vi "Configure Scripting Plugins.vi"() -> ()   [LabVIEW 2016]
uses:
  DQMH Scripting Plugins/PantherLAB Scripting Hooks/Controls or Constants--enum.ctl
  <resource>/dialog/lvconfig.llb/LV Config Read Boolean.vi
  <resource>/dialog/lvconfig.llb/LV Config Read Numeric (I32).vi
  <resource>/dialog/lvconfig.llb/LV Config Write Boolean.vi
  <resource>/dialog/lvconfig.llb/LV Config Write Numeric (I32).vi
  DQMH Scripting Plugins/PantherLAB Scripting Hooks/PantherLAB_Scripting.lvlib
panel:
  in  "wait for reply and timed out? terminals":bool
  in  "Create":T1
  in  "Create Controls/Indicators or Constants":bool
  in  "Panther Logs":bool
  # "If Enabled a fille called <PantherLAB_Log.csv> will be created next to the Active Project and a new row will be logged for all of these DQMH Actions:\n* Add New DQMH Module\n* Rename DQMH Module\n* Duplicate DQMH Module\n* Create New DQMH Event\n* Convert DQMH Event\n* Remove DQMH Event\n* Rename DQMH Event\n* Duplicate DQMH Event\n* Add Helper Looop to DQMH Module\n* Create RT Tester\n* New DQMH Unit Test"
  # "When the DQMH Framework creates a new DQMH Event, it automatically opens the Module's API Tester Block Diagram and it will add the 'Fire Event.vi'  for the new Event Created\n\nTo improve  the process of testing public events, this plugin will create controls and indicators or constants for every public request. You can also choose to include/Exclude the 'wait for reply (T)' and 'timed out?'"
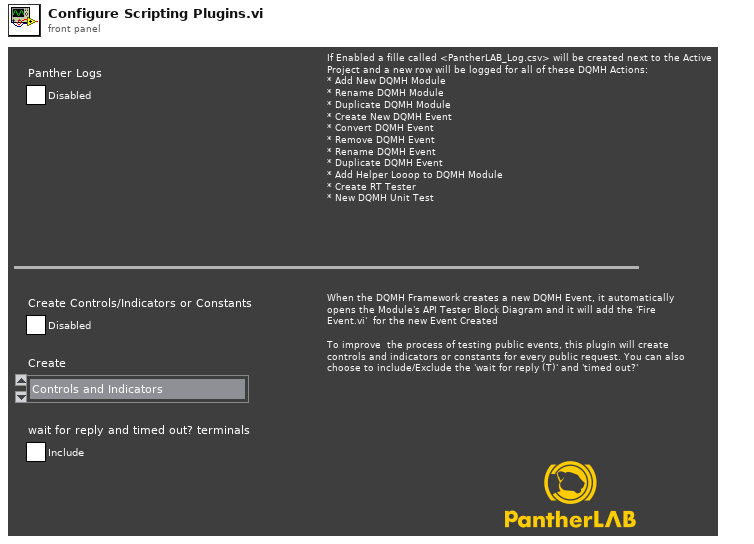
[diagram p1: front panel]
types:
  T1 = typedef "PantherLAB_Scripting.lvlib/Controls or Constants--enum.ctl" = enum16{"Controls and Indicators", "Constants and Indicators"}
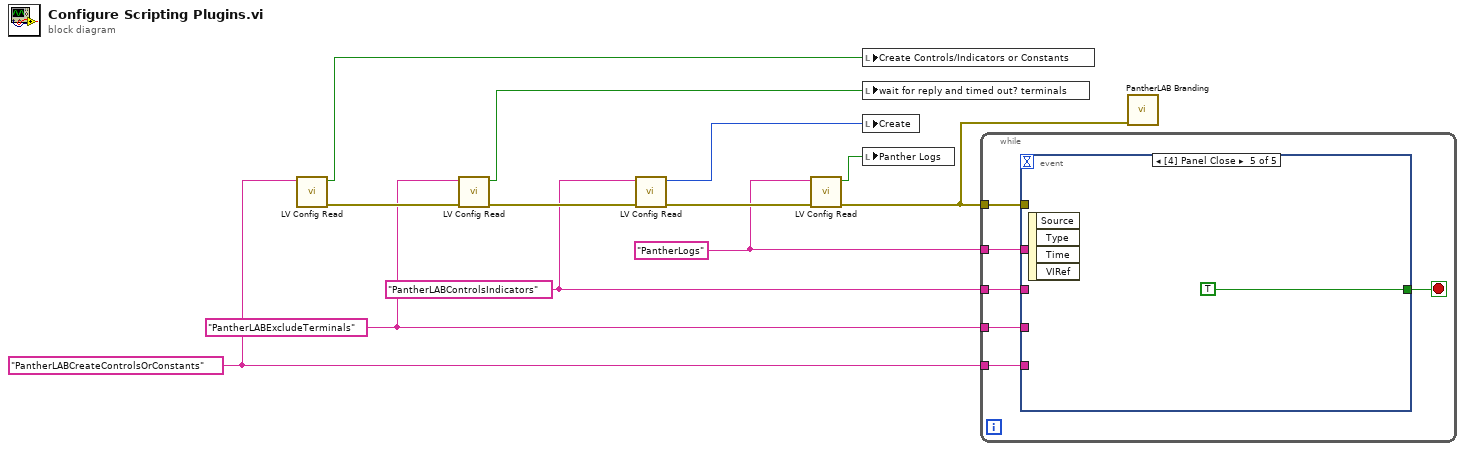
[diagram p0: block diagram]
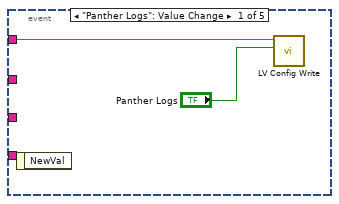
[diagram p2: hidden frame]
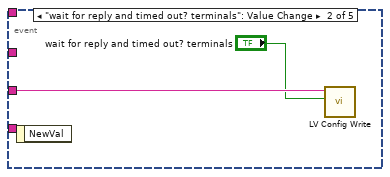
[diagram p3: hidden frame]
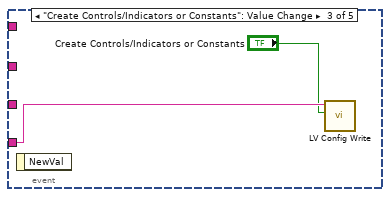
[diagram p4: hidden frame]
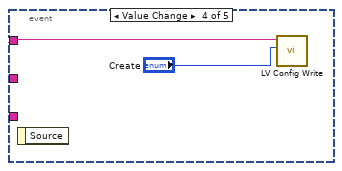
[diagram p5: hidden frame]
diagram:
  w2 = "PantherLABCreateControlsOrConstants" ("key")
  w3 = "PantherLABExcludeTerminals" ("key")
  w1 = "PantherLABControlsIndicators" ("key")
  w4 = "PantherLogs" ("key")
  n1 = call-poly <resource>:"LV Config Read.vi"("key"=w2) -> ("error out"=w10:errorcluster, "value"=w5:bool)  [unwired: 4 in, 1 out]
  n2 = call-poly <resource>:"LV Config Read.vi"("error in"=w10, "key"=w3) -> ("error out"=w11:errorcluster, "value"=w6:bool)  [unwired: 3 in, 1 out]
  n3 = call-poly <resource>:"LV Config Read.vi"("error in"=w11, "key"=w1) -> ("error out"=w12:errorcluster, "value"=w7:i32)  [unwired: 3 in, 1 out]
  n4 = call-poly <resource>:"LV Config Read.vi"("error in"=w12, "key"=w4) -> ("error out"=w9:errorcluster, "value"=w8:bool)  [unwired: 3 in, 1 out]
  n5 = local write "Create Controls/Indicators or Constants"(w5) -> ()
  n6 = local write "wait for reply and timed out? terminals"(w6) -> ()
  n7 = local write "Create"(w7) -> ()
  n8 = local write "Panther Logs"(w8) -> ()
  n9 = while {
    tunnel: w9 -> [w18]
    tunnel: w4 -> [w17]
    tunnel: w3 -> [w16]
    tunnel: w2 -> [w15]
    tunnel: w1 -> [w14]
    stop <- w13 stop-if-true
    n10 = event shown="[4] Panel Close" {
      selector: _ -> [_ _ _ _ _]
      dyn-events: _ -> [_ _ _ _ _]
      timeout: _ -> [_ _ _ _ _]
      tunnel: w18 -> [_ _ _ _ _]
      tunnel: w17 -> [w19 _ _ _ _]
      tunnel: w16 -> [_ w22 _ _ _]
      tunnel: w15 -> [_ _ w24 _ _]
      tunnel: w14 -> [_ _ _ w26 _]
      tunnel: [_ _ _ _ TRUE] -> w13
      event "Panther Logs": Value Change {
        n11 = event-data() -> ()  [unwired: 1 in, 1 out]
        n12 = call-poly <resource>:"LV Config Write.vi"("value"="Panther Logs", "key"=w19) -> ()  [unwired: 5 in, 1 out]
      }
      event "wait for reply and timed out? terminals": Value Change {
        n13 = event-data() -> ()  [unwired: 1 in, 1 out]
        n14 = call-poly <resource>:"LV Config Write.vi"("value"="wait for reply and timed out? terminals", "key"=w22) -> ()  [unwired: 5 in, 1 out]
      }
      event "Create Controls/Indicators or Constants": Value Change {
        n15 = event-data() -> ()  [unwired: 1 in, 1 out]
        n16 = call-poly <resource>:"LV Config Write.vi"("value"="Create Controls/Indicators or Constants", "key"=w24) -> ()  [unwired: 5 in, 1 out]
      }
      event Value Change {
        n17 = event-data() -> ()  [unwired: 1 in, 1 out]
        n18 = call-poly <resource>:"LV Config Write.vi"("value"="Create", "key"=w26) -> ()  [unwired: 5 in, 1 out]
      }
      event Panel Close {
        n19 = event-data() -> ()  [unwired: 1 in, 4 out]
      }
    }
  }
  n20 = call "PantherLAB Branding.vi"("error in"=w9) -> ()  [unwired: 11 in]
